vi "FL Integrate Rule.vi"(7 "integration option":u16(ring) items=["Check rule only", "Add if no conflicts", "Add if partial conflicts", "Replace if full conflict"], 8 "error in (no error)":errorcluster, 9 "new rule":T1 {"consequents"."Var Index" min=0; "consequents"."Cond" items=["=", "!="]; "consequents"."MF Index" min=0; "antecedents"."Var Index" min=0; "antecedents"."Cond" items=["=", "!="]; "antecedents"."MF Index" min=0; "consequent implication" items=["Minimum", "Product"]; "antecedent connective" items=["AND (Minimum)", "AND (Product)", "OR (Maximum)", "OR (Probabilistic)"]}, 11 "fuzzy system in":T7 {"user MF interpolating polynomials"."coa_x(y) coeff" format="%.4g"; "user MF interpolating polynomials"."Area(y) coeff" format="%.4g"; "user MF interpolating polynomials"."X(y) coeff" format="%.4g"; "user MF interpolating polynomials"."Y(x) coeff" format="%.4g"; "user MF interpolating polynomials"."Y" format="%.4g"; "user MF interpolating polynomials"."X" format="%.4g"; "defuzzification method" items=["Center of Area", "Modified Center of Area", "Center of Sums", "Center of Maximum", "Mean of Maximum"]; "rules"."consequents"."Var Index" min=0; "rules"."consequents"."Cond" items=["=", "!="]; "rules"."consequents"."MF Index" min=0; "rules"."antecedents"."Var Index" min=0; "rules"."antecedents"."Cond" items=["=", "!="]; "rules"."antecedents"."MF Index" min=0; "rules"."consequent implication" items=["Minimum", "Product"]; "rules"."antecedent connective" items=["AND (Minimum)", "AND (Product)", "OR (Maximum)", "OR (Probabilistic)"]; "output variables"."MFs"."shape" items=["Triangle", "Trapezoid", "Singleton", "Sigmoid", "Gaussian", "User-Defined"]; "input variables"."MFs"."shape" items=["Triangle", "Trapezoid", "Singleton", "Sigmoid", "Gaussian", "User-Defined"]}) -> (0 "error out":errorcluster, 1 "full rule conflicts":i32[](array[numeric]), 2 "all rule conflicts":i32[](array[numeric]), 3 "fuzzy system out":T7 {"user MF interpolating polynomials"."coa_x(y) coeff" format="%.4g"; "user MF interpolating polynomials"."Area(y) coeff" format="%.4g"; "user MF interpolating polynomials"."X(y) coeff" format="%.4g"; "user MF interpolating polynomials"."Y(x) coeff" format="%.4g"; "user MF interpolating polynomials"."Y" format="%.4g"; "user MF interpolating polynomials"."X" format="%.4g"; "defuzzification method" items=["Center of Area", "Modified Center of Area", "Center of Sums", "Center of Maximum", "Mean of Maximum"]; "rules"."consequents"."Var Index" min=0; "rules"."consequents"."Cond" items=["=", "!="]; "rules"."consequents"."MF Index" min=0; "rules"."antecedents"."Var Index" min=0; "rules"."antecedents"."Cond" items=["=", "!="]; "rules"."antecedents"."MF Index" min=0; "rules"."consequent implication" items=["Minimum", "Product"]; "rules"."antecedent connective" items=["AND (Minimum)", "AND (Product)", "OR (Maximum)", "OR (Probabilistic)"]; "output variables"."MFs"."shape" items=["Triangle", "Trapezoid", "Singleton", "Sigmoid", "Gaussian", "User-Defined"]; "input variables"."MFs"."shape" items=["Triangle", "Trapezoid", "Singleton", "Sigmoid", "Gaussian", "User-Defined"]})   [LabVIEW 2017]
doc: "Checks a new rule for conflicts with existing rules in the fuzzy system and, optionally, integrates the new rule into the system."
uses:
  <vilib>/addons/Fuzzy Logic/TypeDefs/FL System.ctl
  <vilib>/addons/Fuzzy Logic/TypeDefs/FL Variable.ctl
  <vilib>/addons/Fuzzy Logic/TypeDefs/FL Membership Function.ctl
  <vilib>/addons/Fuzzy Logic/TypeDefs/FL Membership Function Shape.ctl
  <vilib>/addons/Fuzzy Logic/TypeDefs/FL Rule.ctl
  <vilib>/addons/Fuzzy Logic/TypeDefs/FL Antecedent.ctl
  <vilib>/addons/Fuzzy Logic/TypeDefs/FL Modifier.ctl
  <vilib>/addons/Fuzzy Logic/TypeDefs/FL Antecedent Connective.ctl
  <vilib>/addons/Fuzzy Logic/TypeDefs/FL Consequent.ctl
  <vilib>/addons/Fuzzy Logic/TypeDefs/FL Consequent Implication.ctl
  <vilib>/addons/Fuzzy Logic/TypeDefs/FL Defuzzification.ctl
  <vilib>/addons/Fuzzy Logic/TypeDefs/FL Interpolating polynomials.ctl
  <vilib>/addons/Fuzzy Logic/NI_Fuzzy_Logic_API.lvlib
panel:
  # "IF"
  # "THEN"
  # "IF"
  # "THEN"
  # "IF"
  # "THEN"
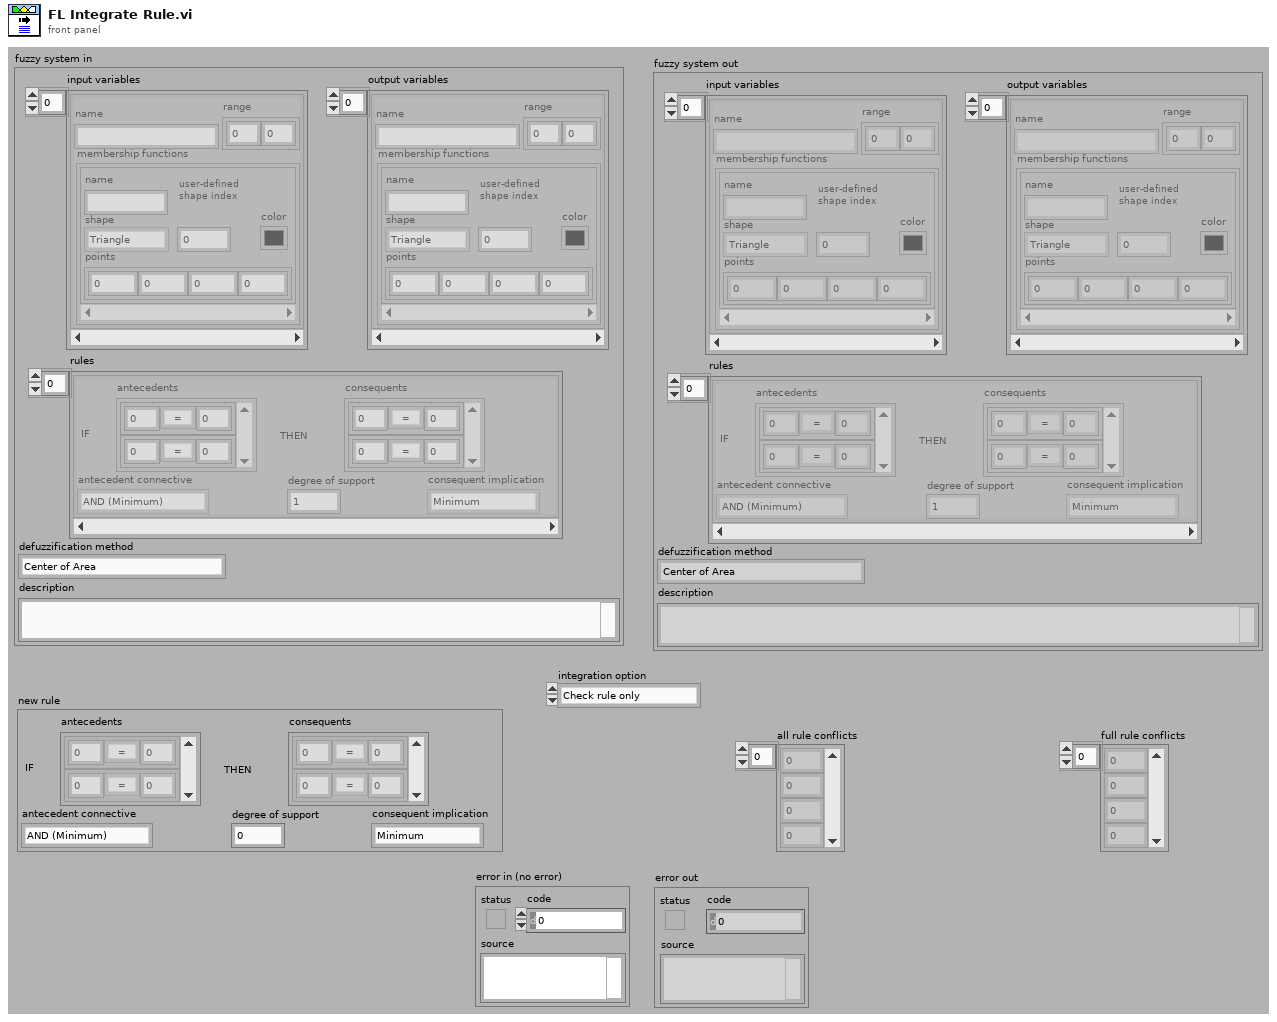
[diagram p1: front panel]
types:
  T1 = typedef "NI_Fuzzy_Logic_API.lvlib/FL Rule.ctl" = cluster{"antecedents":T2[], "antecedent connective":T4, "consequents":T5[], "consequent implication":T6, "degree of support":dbl}
  T2 = typedef "NI_Fuzzy_Logic_API.lvlib/FL Antecedent.ctl" = cluster{"Var Index":i32, "MF Index":i32, "Cond":T3}
  T3 = typedef "NI_Fuzzy_Logic_API.lvlib/FL Modifier.ctl" = u16
  T4 = typedef "NI_Fuzzy_Logic_API.lvlib/FL Antecedent Connective.ctl" = u16
  T5 = typedef "NI_Fuzzy_Logic_API.lvlib/FL Consequent.ctl" = cluster{"Var Index":i32, "MF Index":i32, "Cond":T3}
  T6 = typedef "NI_Fuzzy_Logic_API.lvlib/FL Consequent Implication.ctl" = u16
  T7 = typedef "NI_Fuzzy_Logic_API.lvlib/FL System.ctl" = cluster{"input variables":T8[], "output variables":T8[], "rules":T1[], "defuzzification method":T11, "description":string, "user MF interpolating polynomials":T12[]}
  T8 = typedef "NI_Fuzzy_Logic_API.lvlib/FL Variable.ctl" = cluster{"name":string, "range":dbl[], "MFs":T9[]}
  T9 = typedef "NI_Fuzzy_Logic_API.lvlib/FL Membership Function.ctl" = cluster{"name":string, "shape":T10, "points":dbl[], "color":u32, "user-defined shape index":i32}
  T10 = typedef "NI_Fuzzy_Logic_API.lvlib/FL Membership Function Shape.ctl" = u16
  T11 = typedef "NI_Fuzzy_Logic_API.lvlib/FL Defuzzification.ctl" = u16
  T12 = typedef "NI_Fuzzy_Logic_API.lvlib/FL Interpolating polynomials.ctl" = cluster{"X":dbl[], "Y":dbl[], "Y(x) coeff":dbl[][], "X(y) coeff":dbl[][], "Area(y) coeff":dbl[][], "coa_x(y) coeff":dbl[][]}
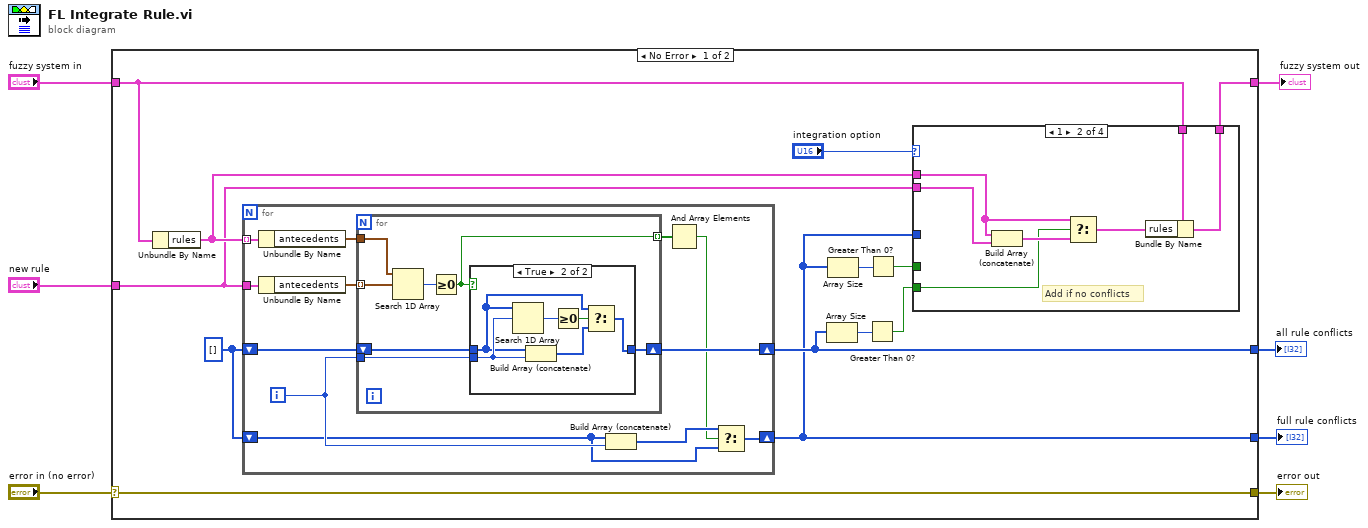
[diagram p0: block diagram]
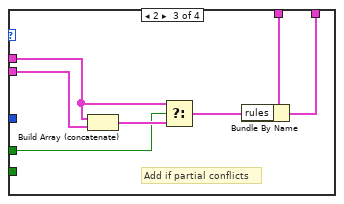
[diagram p3: hidden frame]
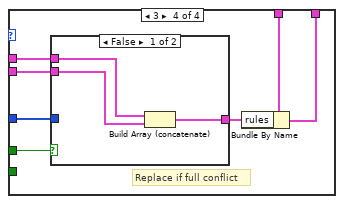
[diagram p4: hidden frame]
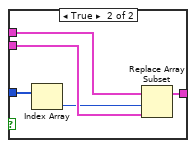
[diagram p5: hidden frame]
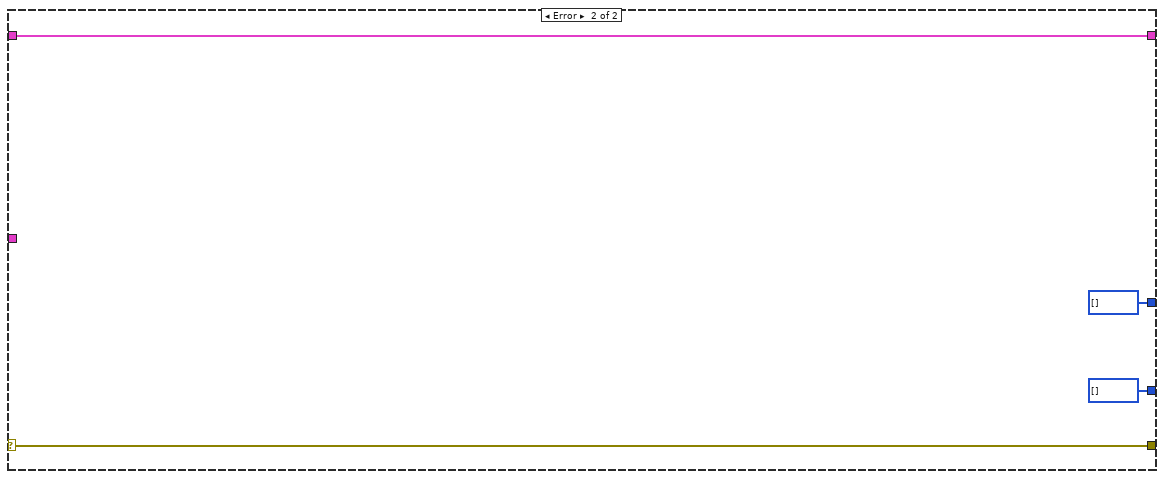
[diagram p7: hidden frame]
diagram:
  n1 = case shown="No Error" "error in (no error)" {
    selector: "error in (no error)" -> [w8 w77]
    tunnel: "new rule" -> [w19 _]
    tunnel: [w18 i32[] []] -> w6
    tunnel: [w17 w80] -> w5
    tunnel: "fuzzy system in" -> [w16 w80]
    tunnel: [w9 i32[] []] -> w3
    tunnel: [w8 w77] -> w1
    frame No Error {
      w12 = i32[] []
      n2 = Unbundle By Name(w16) -> ("rules"=w20:T1[])
      n3 = for {
        tunnel: w20 -> [w62] mode=indexing
        tunnel: w19 -> [w61]
        shift-right: [w57] -> w18
        shift-left: w12 -> [w58]
        shift-right: [w55] -> w9
        shift-left: w12 -> [w51]
        i -> [w54]
        n4 = Unbundle By Name(w62) -> ("antecedents"=w60:T2[])
        n5 = Unbundle By Name(w61) -> ("antecedents"=w59:T2[])
        n6 = for {
          tunnel: w60 -> [w69]
          tunnel: w59 -> [w68] mode=indexing
          tunnel: w54 -> [w65]
          shift-right: [w64] -> w57
          shift-left: w58 -> [w66]
          tunnel: [w63] -> w56 mode=indexing
          n7 = Search 1D Array(1D array=w69, element=w68) -> (index of element=w67:i32)  [unwired: 1 in]
          n8 = Greater Or Equal To 0?(x=w67) -> (x >= 0?=w63:bool)
          n9 = case shown="True" w63 {
            tunnel: w66 -> [w70 w73]
            tunnel: w65 -> [_ w76]
            tunnel: [w70 w71] -> w64
            frame False {
            }
            frame True {
              n10 = Search 1D Array(1D array=w73, element=w76) -> (index of element=w75:i32)  [unwired: 1 in]
              n11 = Build Array (concatenate)(w73, w76) -> (w72:i32[])
              n12 = Greater Or Equal To 0?(x=w75) -> (x >= 0?=w74:bool)
              n13 = Select(t=w73, s=w74, f=w72) -> (s? t:f=w71:i32[])
            }
          }
        }
        n14 = Build Array (concatenate)(w51, w54) -> (w53:i32[])
        n15 = And Array Elements(Boolean array=w56) -> (logical AND=w52:bool)
        n16 = Select(t=w53, s=w52, f=w51) -> (s? t:f=w55:i32[])
      }
      n17 = Array Size(array=w18) -> (size(s)=w14:i32)
      n18 = Array Size(array=w9) -> (size(s)=w11:i32)
      n19 = Greater Than 0?(x=w14) -> (x > 0?=w13:bool)
      n20 = Greater Than 0?(x=w11) -> (x > 0?=w10:bool)
      n21 = case shown="1" "integration option" {
        tunnel: w13 -> [_ w22 _ _]
        tunnel: [w21 w27 w34 w41] -> w17
        tunnel: w16 -> [w21 w28 w35 w42]
        tunnel: w20 -> [_ w25 w32 w40]
        tunnel: w19 -> [_ w26 w33 w39]
        tunnel: w10 -> [_ _ w29 w36]
        tunnel: w9 -> [_ _ _ w37]
        frame 0, Default {
          # "Check rule only"
        }
        frame 1 {
          # "Add if no conflicts"
          n22 = Build Array (concatenate)(w25, w26) -> (w24:T1[])
          n23 = Select(t=w25, s=w22, f=w24) -> (s? t:f=w23:T1[])
          n24 = Bundle By Name(cluster=w28, "rules"=w23) -> (w27:T7)
        }
        frame 2 {
          # "Add if partial conflicts"
          n25 = Build Array (concatenate)(w32, w33) -> (w31:T1[])
          n26 = Select(t=w32, s=w29, f=w31) -> (s? t:f=w30:T1[])
          n27 = Bundle By Name(cluster=w35, "rules"=w30) -> (w34:T7)
        }
        frame 3 {
          # "Replace if full conflict"
          n28 = case shown="False" w36 {
            tunnel: w40 -> [w45 w50]
            tunnel: w39 -> [w44 w49]
            tunnel: [w43 w48] -> w38
            tunnel: w37 -> [_ w47]
            frame False {
              n29 = Build Array (concatenate)(w45, w44) -> (w43:T1[])
            }
            frame True {
              n30 = Index Array(array=w47) -> (element=w46:i32)  [unwired: 1 in]
              n31 = Replace Array Subset(array=w50, new element=w49, index=w46) -> (w48:T1[])
            }
          }
          n32 = Bundle By Name(cluster=w42, "rules"=w38) -> (w41:T7)
        }
      }
    }
    frame Error {
    }
  }
  "fuzzy system out" <- w5
  "all rule conflicts" <- w6
  "full rule conflicts" <- w3
  "error out" <- w1
